vi "Show Event.vi"(8 "error in (no error)":errorcluster, 10 "Panel":string) -> (0 "error out":errorcluster)   [LabVIEW 2023, in "Panel Actor.lvlib" / "Panel.lvlib" / "Panel Registry.lvclass"]
doc: "If all ancestors of the panel are shown, then broadcasts a \"Shown\" Panel event to all of the panels children.\n\nIf one of the ancestors isn't shown, then no events are broadcast.\n\n----\nPlease see the following web address for additional documentation and tutorial information:\nhttp://www.mooregoodideas.com/mgi-panel-manager/\n\nAuthor: Derek Trepanier\n\nCopyright (c) 2018, Moore Good Ideas, Inc.\n\nAll rights reserved.\n\nRedistribution and use in source and binary forms, with or without modification, are permitted provided that the following conditions are met:\n\n * Redistributions of source code must retain the above copyright notice, this list of conditions and the following disclaimer.\n * Redistributions in binary form must reproduce the above copyright notice, this list of conditions and the following disclaimer in the documentation and/or other materials provided with the distribution.\n * Neither the name of Moore Good Ideas, Inc. nor the names of its contributors may be used to endorse or promote products derived from this software without specific prior written permission.\n\nTHIS SOFTWARE IS PROVIDED BY THE COPYRIGHT HOLDERS AND CONTRIBUTORS \"AS IS\" AND ANY EXPRESS OR IMPLIED WARRANTIES, INCLUDING, BUT NOT LIMITED TO, THE IMPLIED WARRANTIES OF MERCHANTABILITY AND FITNESS FOR A PARTICULAR PURPOSE ARE DISCLAIMED. IN NO EVENT SHALL THE COPYRIGHT OWNER OR CONTRIBUTORS BE LIABLE FOR ANY DIRECT, INDIRECT, INCIDENTAL, SPECIAL, EXEMPLARY, OR CONSEQUENTIAL DAMAGES (INCLUDING, BUT NOT LIMITED TO, PROCUREMENT OF SUBSTITUTE GOODS OR SERVICES; LOSS OF USE, DATA, OR PROFITS; OR BUSINESS INTERRUPTION) HOWEVER CAUSED AND ON ANY THEORY OF LIABILITY, WHETHER IN CONTRACT, STRICT LIABILITY, OR TORT (INCLUDING NEGLIGENCE OR OTHERWISE) ARISING IN ANY WAY OUT OF THE USE OF THIS SOFTWARE, EVEN IF ADVISED OF THE POSSIBILITY OF SUCH DAMAGE."
uses:
  Panel Registry.lvclass
  Panel Registry.lvclass/Panel Registry.ctl
  Panel Helper/Events.ctl
  Panel Helper/Panel Helper.lvclass
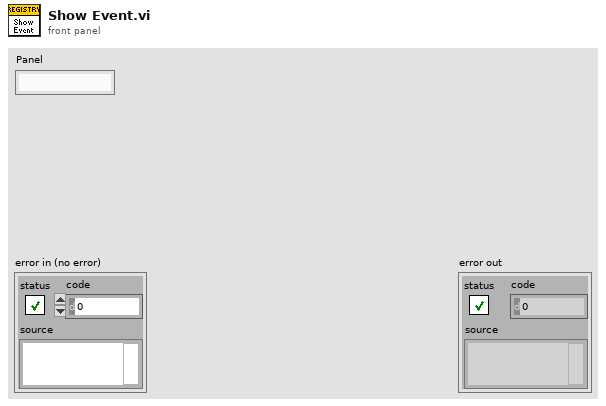
[diagram p1: front panel]
types:
  T1 = typedef "Panel Actor.lvlib/Panel.lvlib/Panel Helper.lvclass/Events.ctl" = enum16{"Initialized", "Shown", "Hidden", "Closed"}
  T2 = enum32{"Invalid", "Standard", "Closed", "Hidden", "Minimized", "Maximized"}
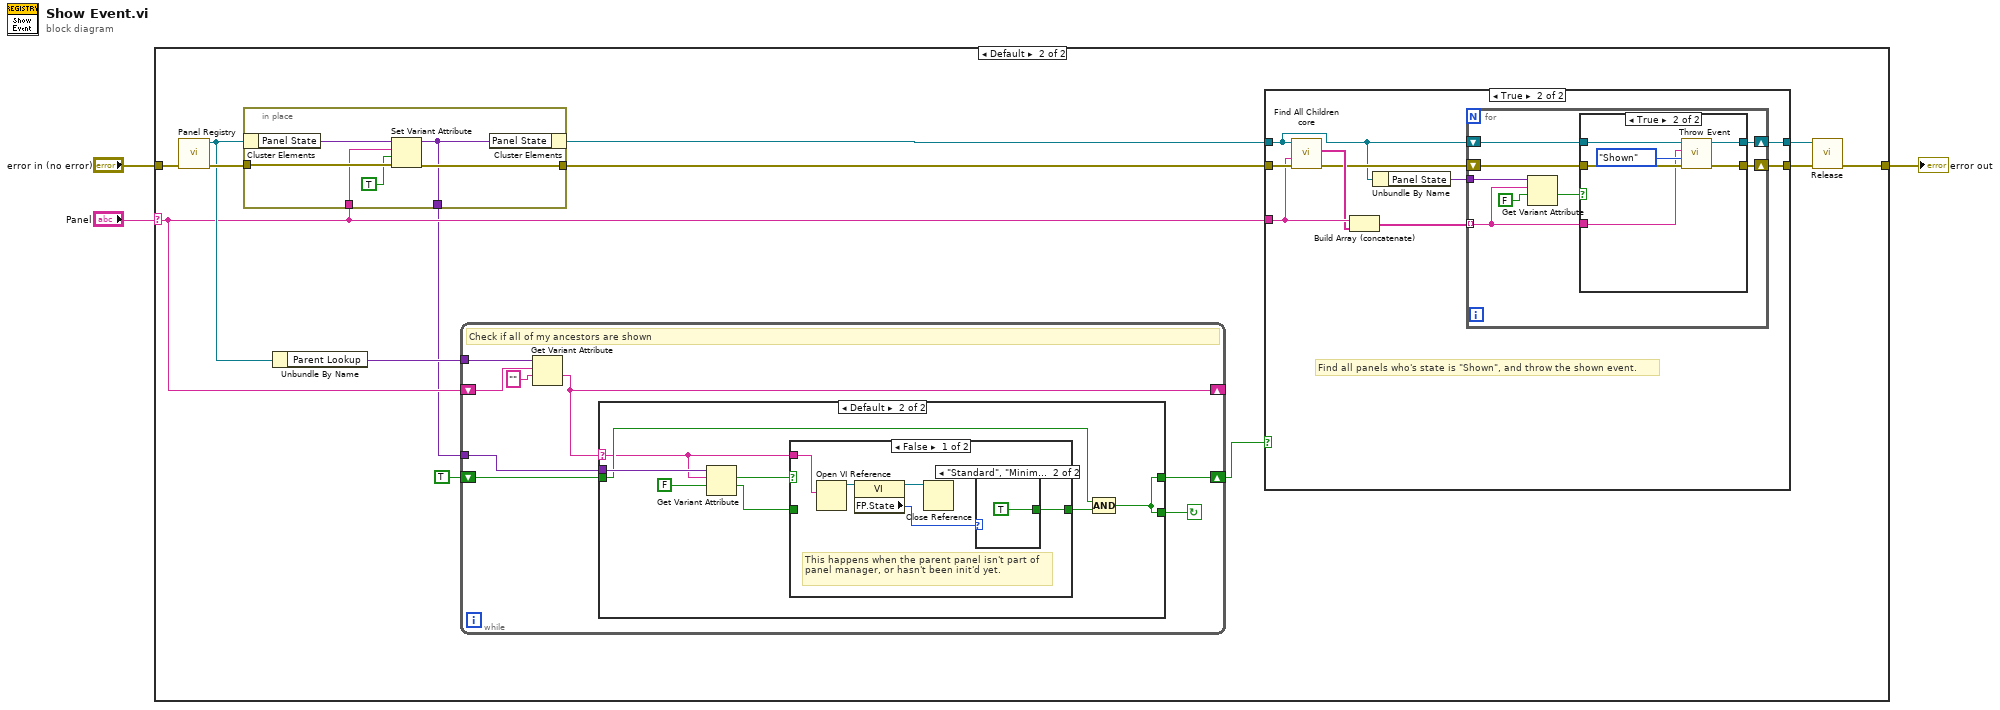
[diagram p0: block diagram]
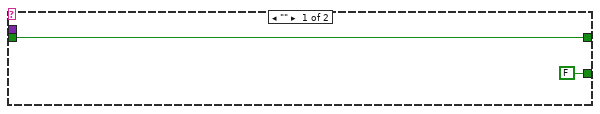
[diagram p5: hidden frame]
diagram:
  n1 = case shown="Default" "Panel" {
    selector: "Panel" -> [_ w10]
    tunnel: "error in (no error)" -> [w4 w17]
    tunnel: [w4 w16] -> w2
    frame "" {
    }
    frame Default {
      n2 = call "Panel Registry.vi"("error in (no error)"=w17) -> ("error out"=w14:errorcluster, "Panel Registry out"=w12:refnum<class "Panel Registry.lvclass">)  [unwired: 9 in]
      n3 = in-place {
        in-place-border: w14 -> [w22]
        in-place-border: w10 -> [w21]
        in-place-border: [w20] -> w6
        in-place-border: [w18] -> w5
        n4 = in-place-cluster #1(w12) -> ("Panel State"=w23:variant)
        n5 = Set Variant Attribute(Variant=w23, name=w21, value=TRUE, error in=w22) -> (Variant out=w18:variant, error out=w20:errorcluster)  [unwired: 1 out]
        n6 = in-place-cluster #1("Panel State"=w18) -> (w7:refnum<class "Panel Registry.lvclass">)
      }
      n7 = Unbundle By Name(w12) -> ("Parent Lookup"=w15:variant)
      n8 = while {
        shift-right: [w54] -> _
        shift-left: w10 -> [w57]
        tunnel: w15 -> [w58]
        tunnel: w5 -> [w55]
        shift-right: [w52] -> w8
        shift-left: TRUE -> [w53]
        stop <- w51 continue-if-true
        # "Check if all of my ancestors are shown"
        n9 = Get Variant Attribute(Variant=w58, name=w57, default value (empty Variant)="" ("VI")) -> (value=w54:string)  [unwired: 1 in, 3 out]
        n10 = case shown="Default" w54 {
          selector: w54 -> [_ w63]
          tunnel: w55 -> [_ w68]
          tunnel: w53 -> [w60 w67]
          tunnel: [w60 w66] -> w52
          tunnel: [FALSE w66] -> w51
          frame "" {
          }
          frame Default {
            n11 = Get Variant Attribute(Variant=w68, name=w63, default value (empty Variant)=FALSE) -> (found=w65:bool, value=w61:bool)  [unwired: 1 in, 2 out]
            n12 = case shown="False" w65 {
              tunnel: [w69 w75] -> w64
              tunnel: w61 -> [_ w75]
              tunnel: w63 -> [w73 _]
              frame False {
                # "This happens when the parent panel isn't part of panel manager, or hasn't been init'd yet."
                n13 = Open VI Reference(vi path=w73) -> (vi reference=w72:refnum<vi>)  [unwired: 5 in, 1 out]
                n14 = property class="VI"(reference=w72) -> (reference out=w71:refnum<vi>, "FP.State"=w70:T2)  [unwired: 1 in, 1 out]
                n15 = Close Reference(reference=w71) -> ()  [unwired: 1 in, 1 out]
                n16 = case shown="\"Standard\", \"Minimized\", \"Maximized\"" w70 {
                  tunnel: [_ TRUE] -> w69
                  frame Default {
                  }
                  frame "Standard", "Minimized", "Maximized" {
                  }
                }
              }
              frame True {
              }
            }
            n17 = Compound Arithmetic op=AND(w67, w64) -> (w66:bool)
          }
        }
      }
      n18 = case shown="True" w8 {
        tunnel: w6 -> [w24 w34]
        tunnel: w7 -> [w25 w27]
        tunnel: [w24 w28] -> w13
        tunnel: w10 -> [_ w33]
        tunnel: [w25 w29] -> w11
        frame False {
        }
        frame True {
          # "Find all panels who's state is \"Shown\", and throw the shown event."
          n19 = call "Find All Children core.vi"("error in (no error)"=w34, "Panel"=w33, "Panel Registry in"=w27) -> ("error out"=w31:errorcluster, "All Children"=w32:string[])  [unwired: 7 in]
          n20 = Build Array (concatenate)(w33, w32) -> (w30:string[])
          n21 = Unbundle By Name(w27) -> ("Panel State"=w26:variant)
          n22 = for {
            shift-right: [w39] -> w28
            shift-left: w31 -> [w42]
            tunnel: w30 -> [w37] mode=indexing
            shift-right: [w41] -> w29
            shift-left: w27 -> [w40]
            tunnel: w26 -> [w38]
            n23 = Get Variant Attribute(Variant=w38, name=w37, default value (empty Variant)=FALSE) -> (value=w35:bool)  [unwired: 1 in, 3 out]
            n24 = case shown="True" w35 {
              tunnel: w42 -> [w43 w50]
              tunnel: [w44 w49] -> w41
              tunnel: w40 -> [w44 w48]
              tunnel: [w43 w47] -> w39
              tunnel: w37 -> [_ w45]
              frame False {
              }
              frame True {
                n25 = call "Throw Event.vi"("error in (no error)"=w50, "Event"=Events."Shown", "Panel"=w45, "Panel Registry in"=w48) -> ("error out"=w47:errorcluster, "Panel Registry out"=w49:refnum<class "Panel Registry.lvclass">)  [unwired: 6 in]
              }
            }
          }
        }
      }
      n26 = call "Release.vi"("error in (no error)"=w13, "Panel Registry in"=w11) -> ("error out"=w16:errorcluster)  [unwired: 9 in]
    }
  }
  "error out" <- w2
